vi "InitFromXML.vi"(8 "error in (no error)":errorcluster, 10 "XML":string, 11 "Web in":refnum<class "Web.lvclass">) -> (0 "error out":errorcluster, 3 "Web out":refnum<class "Web.lvclass">)   [LabVIEW 2009, in "NavScreen.lvlib" / "Web.lvclass"]
uses:
  Web.lvclass
  ClickableText/ClickableText.lvclass
  Web.lvclass/Web.ctl
  NavScreen.lvlib
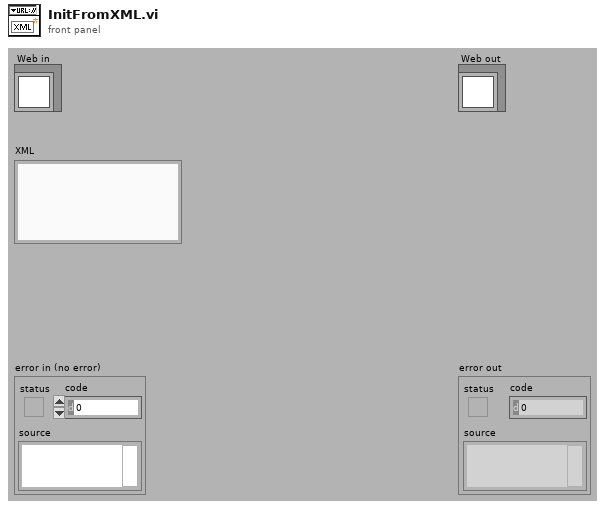
[diagram p1: front panel]
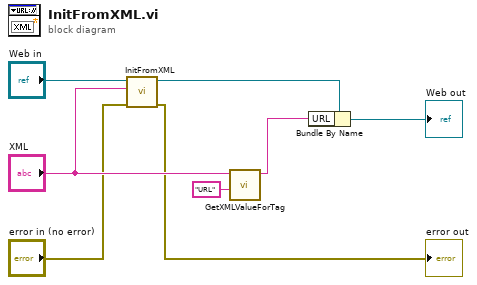
[diagram p0: block diagram]
diagram:
  n1 = call-parent "InitFromXML.vi"("error in (no error)"="error in (no error)", "XML"="XML", "ClickableText in"="Web in") -> ("error out"=→"error out":errorcluster, "ClickableText out"=w8:refnum<class "Web.lvclass">)  [unwired: 7 in]
  n2 = call "GetXMLValueForTag.vi"("tag"="URL", "XML"="XML") -> ("value"=w2:string)  [unwired: 8 in, 1 out]
  n3 = Bundle By Name(cluster=w8, "URL"=w2) -> (→"Web out":refnum<class "Web.lvclass">)
